vi "AllocateArray.vi"(3 "URAPI in":string) -> (1 "URAPI out":string)   [LabVIEW 2012]
panel:
  out "reversed":string
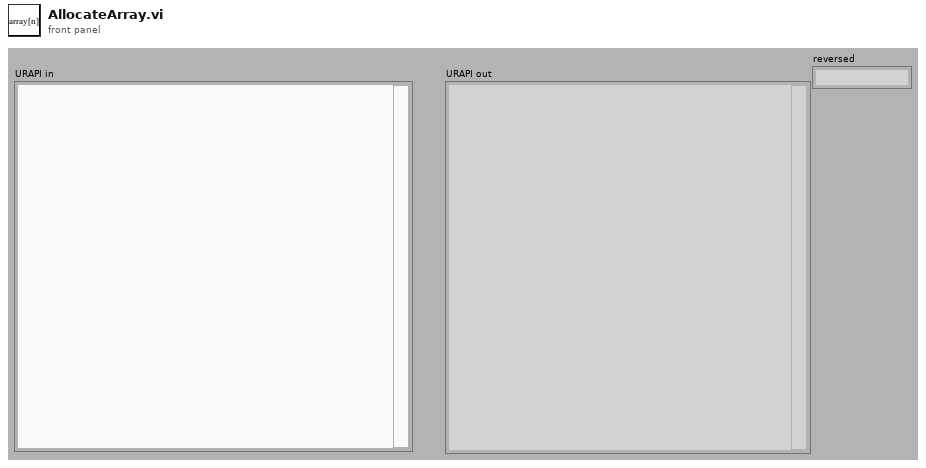
[diagram p1: front panel]
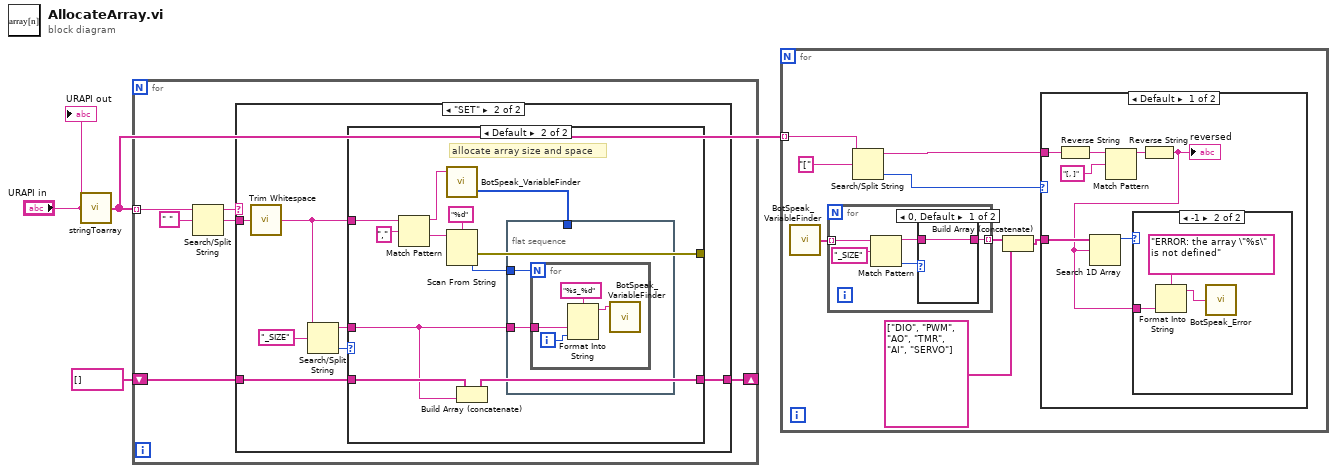
[diagram p0: block diagram]
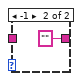
[diagram p2: hidden frame]
diagram:
  n1 = call <userlib>:"stringToarray.vi"("String"="URAPI in") -> ("Array"=w2:string[])
  n2 = for {
    tunnel: w2 -> [w7] mode=indexing
    shift-right: [w5] -> _
    shift-left: string[] [] -> [w4]
    n3 = Search/Split String(string=w7, search string/char (-)=" ") -> (substring before match=w8:string, match + rest of string=w6:string)  [unwired: 1 in, 1 out]
    n4 = case shown="\"SET\"" w8 {
      tunnel: w6 -> [_ w14]
      tunnel: [w10 w13] -> w5
      tunnel: w4 -> [w10 w12]
      frame Default {
      }
      frame "SET" {
        n5 = call <vilib>:"Trim Whitespace.vi"("string"=w14) -> ("trimmed string"=w11:string)  [unwired: 1 in]
        n6 = Search/Split String(string=w11, search string/char (-)="_SIZE") -> (substring before match=w15:string, offset of match=w16:i32)  [unwired: 1 in, 1 out]
        n7 = case shown="Default" w16 {
          tunnel: w15 -> [_ w19]
          tunnel: [_ w27] -> _
          tunnel: w11 -> [_ w24]
          tunnel: [w18 w22] -> w13
          tunnel: w12 -> [w18 w21]
          frame -1 {
          }
          frame Default {
            # "allocate array size and space"
            n8 = Match Pattern(string=w24, regular expression="," ("search string/char (-)")) -> (before substring=w23:string, after substring=w25:string)  [unwired: 1 in, 2 out]
            n9 = call <userlib>:"BotSpeak_VariableFinder.vi"("variable name"=w23) -> ("codes"=w20:u8[])  [unwired: 2 in, 1 out]
            n10 = Scan From String(format string="%d", input string=w25) -> (error out=w27:errorcluster, output 1=w29:i32)  [unwired: 3 in, 2 out]
            n11 = Build Array (concatenate)(w21, w19) -> (w22:string[])
            n12 = flat-sequence {
              tunnel: w29 -> [w31]
              tunnel: w19 -> [w30]
              tunnel: w20 -> [_]
              frame #0 {
                n13 = for {
                  N: w31 -> [_]
                  tunnel: w30 -> [w33]
                  i -> [w32]
                  n14 = Format Into String(format string="%s_%d", w33, w32) -> (resulting string=w35:string)  [unwired: 2 in, 1 out]
                  n15 = call <userlib>:"BotSpeak_VariableFinder.vi"("variable name"=w35) -> ()  [unwired: 2 in, 2 out]
                }
              }
            }
          }
        }
      }
    }
  }
  n16 = for {
    tunnel: w2 -> [w43] mode=indexing
    n17 = call <userlib>:"BotSpeak_VariableFinder.vi"() -> ("Variables"=w39:string[])  [unwired: 3 in, 1 out]
    n18 = for {
      tunnel: w39 -> [w47] mode=indexing
      tunnel: [w45] -> w38 mode=indexing
      n19 = Match Pattern(string=w47, regular expression="_SIZE" ("search string/char (-)")) -> (before substring=w44:string, offset past match=w46:i32)  [unwired: 1 in, 2 out]
      n20 = case shown="0, Default" w46 {
        tunnel: [w49 "" ("Var")] -> w45
        tunnel: w44 -> [w49 _]
        frame 0, Default {
        }
        frame -1 {
        }
      }
    }
    n21 = Search/Split String(string=w43, search string/char (-)="[" ("regular expression")) -> (substring before match=w40:string, offset of match=w41:i32)  [unwired: 1 in, 1 out]
    n22 = Build Array (concatenate)(w38, string[] ["DIO", "PWM", "AO", "TMR", "AI", "SERVO"]) -> (w37:string[])
    n23 = case shown="Default" w41 {
      tunnel: w40 -> [w57 _]
      tunnel: w37 -> [w53 _]
      frame Default {
        n24 = Reverse String(1:w57) -> (0:w56:string)
        n25 = Match Pattern(string=w56, regular expression="[, ]") -> (before substring=w54:string)  [unwired: 1 in, 3 out]
        n26 = Reverse String(1:w54) -> (0:w51:string)
        "reversed" <- w51
        n27 = Search 1D Array(1D array=w53, element=w51) -> (index of element=w52:i32)  [unwired: 1 in]
        n28 = case shown="-1" w52 {
          tunnel: w51 -> [_ w58]
          frame 0, Default {
          }
          frame -1 {
            n29 = Format Into String(format string="ERROR: the array \"%s\" is not defined" ("message"), w58) -> (resulting string=w59:string)  [unwired: 2 in, 1 out]
            n30 = call <userlib>:"BotSpeak_Error.vi"("Error String"=w59) -> ()
          }
        }
      }
      frame -1 {
      }
    }
  }
  "URAPI out" <- "URAPI in"
